vi "KE2260B Reset Output Protection.vi"(8 "error in (no error)":errorcluster, 11 "VISA resource name":refnum<visa-resource-name>) -> (0 "error out":errorcluster, 3 "VISA resource name out":refnum<visa-resource-name>)   [LabVIEW 2021, in "Keithley 2260B.lvlib"]
doc: "Resets the status of over voltage protection (OVP) ,over current protection (OCP), over temperature protection (OTP), and shutdown alarm."
uses:
  Keithley 2260B.lvlib
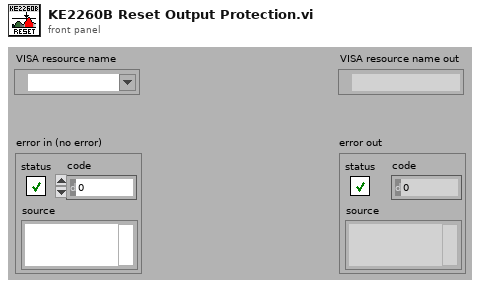
[diagram p1: front panel]
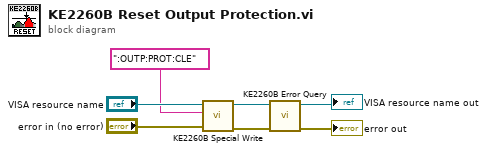
[diagram p0: block diagram]
diagram:
  n1 = call "KE2260B Special Write.vi"("error in (no error)"="error in (no error)", "Write Buffer (\"\")"=":OUTP:PROT:CLE" ("write buffer"), "VISA session"="VISA resource name") -> ("error out"=w3:errorcluster, "dup VISA session"=w4:refnum<visa-resource-name>)  [unwired: 6 in, 1 out]
  n2 = call "KE2260B Error Query.vi"("error in (no error)"=w3, "VISA resource name"=w4) -> ("error out"=→"error out":errorcluster, "VISA resource name out"=→"VISA resource name out":refnum<visa-resource-name>)  [unwired: 6 in, 2 out]
